vi "20170321-lecture3-2 AutoIndex.vi"() -> ()   [LabVIEW 2014]
panel:
  out "Array 3":dbl[][](array[numeric])
  out "Array 2":dbl[][](array[numeric])
  out "Array":dbl[][](array[numeric])
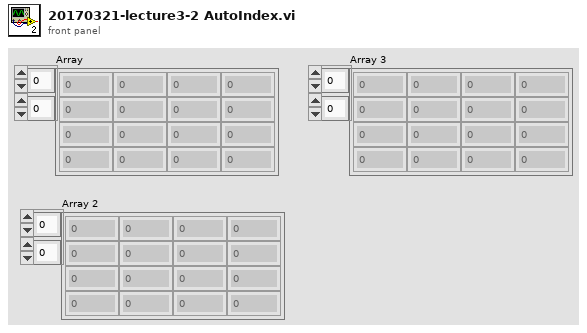
[diagram p1: front panel]
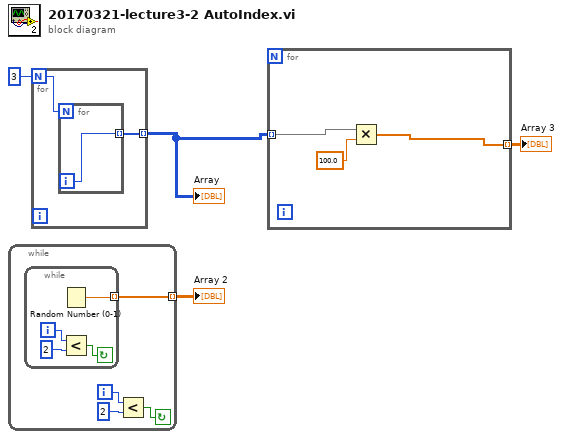
[diagram p0: block diagram]
diagram:
  n1 = while {
    tunnel: [w5] -> w3 mode=indexing
    i -> [w7]
    stop <- w6 continue-if-true
    n2 = while {
      tunnel: [w9] -> w5 mode=indexing
      i -> [w10]
      stop <- w12 continue-if-true
      n3 = Random Number (0-1)() -> (number: 0 to 1=w9:dbl)
      n4 = Less?(x=w10, y=2) -> (x < y?=w12:bool)
    }
    n5 = Less?(x=w7, y=2) -> (x < y?=w6:bool)
  }
  "Array 2" <- w3
  n6 = for {
    N: 3 -> [w13]
    tunnel: [w14] -> w2 mode=indexing
    n7 = for {
      N: w13 -> [_]
      tunnel: [w15] -> w14 mode=indexing
      i -> [w15]
    }
  }
  "Array" <- w2
  n8 = for {
    tunnel: w2 -> [w18] mode=indexing
    tunnel: [w17] -> w1 mode=indexing
    n9 = Multiply(x=w18, y=100.0) -> (x*y=w17:dbl[])
  }
  "Array 3" <- w1
